vi "PathPlanner_PathFinder_ClearIncons.vi"() -> (3 "Incons":map{i32, T1}(c390))   [LabVIEW 2019]
uses:
  PathPlannerLib24/TypeDef/PathPlannerFinderDoublePair.ctl
  PathPlannerLib24/PathPlanner24.lvlib
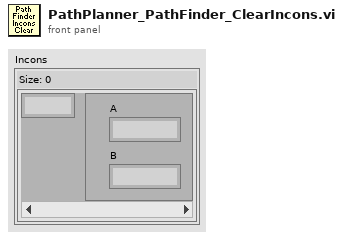
[diagram p1: front panel]
types:
  T1 = typedef "PathPlanner24.lvlib/PathPlannerFinderDoublePair.ctl" = cluster{"A":dbl, "B":dbl}
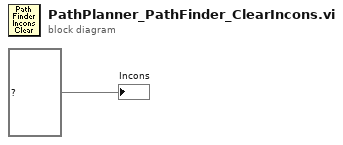
[diagram p0: block diagram]
diagram:
  "Incons" <- map{i32, T1} {} ("Incons")
